vi "Write YSI Data X.vi"(0 "Output File":path=path "c:/junk.dat", 5 "Absolute Depth In":sgl format="%.2f", 7 "Zeroed Pressure":dbl format="%.2f", 9 "YSI Array":dbl[](array[numeric]) format="%.2f", 11 "Update Pressure = False\nUpdate YSI = True":bool) -> ()   [LabVIEW 2016]
uses:
  <vilib>/Utility/file.llb/Read From Spreadsheet File (DBL).vi
  <vilib>/Utility/file.llb/Write To Spreadsheet File (DBL).vi
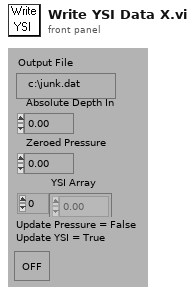
[diagram p1: front panel]
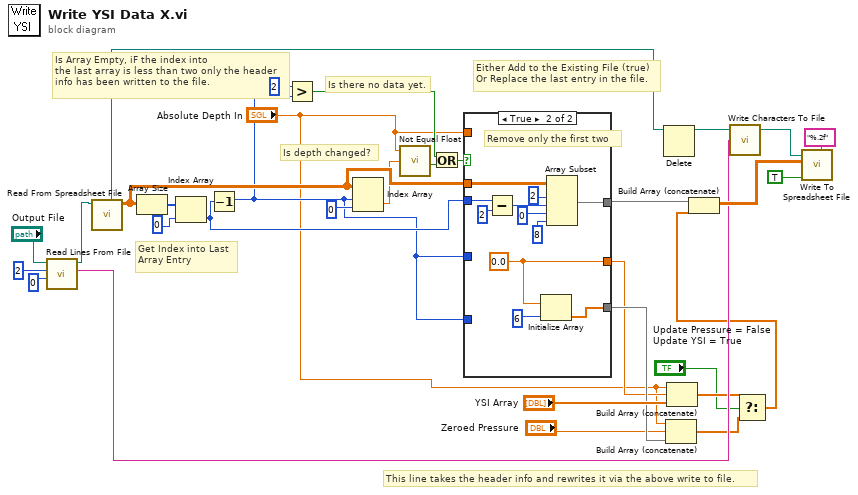
[diagram p0: block diagram]
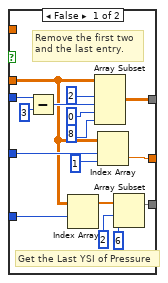
[diagram p2: hidden frame]
diagram:
  # "Is there no data yet."
  # "This line takes the header info and rewrites it via the above write to file."
  # "Either Add to the Existing File (true)\nOr Replace the last entry in the file."
  # "Get Index into Last \nArray Entry"
  # "Is depth changed?"
  # "Is Array Empty, iF the index into\nthe last array is less than two only the header\ninfo has been written to the file."
  n1 = call <vilib>:"Read Lines From File.vi"("file path (dialog if empty)"="Output File", "number of lines (all:-1)"=2, "start of read offset (chars.:0)"=0) -> ("new file path (Not A Path if cancelled)"=w14:path, "line string"=w16:string)  [unwired: 3 in, 2 out]
  n2 = call-poly <vilib>:"Read From Spreadsheet File.vi"("file path (dialog if empty)"=w14) -> ("all rows"=w23:dbl[][], "new file path (Not A Path if cancelled)"=w13:path)  [unwired: 6 in, 3 out]
  n3 = Array Size(array=w23) -> (size(s)=w32:i32[])
  n4 = Index Array(array=w32, index=0) -> (element=w12:i32)
  n5 = Decrement(x=w12) -> (x-1=w11:i32)
  n6 = Greater?(x=2, y=w11) -> (0:w25:bool)
  n7 = Index Array(array=w23, index (row)=w11, index (col)=0) -> (element=w1:dbl)
  n8 = call "Not Equal Float.vi"("Input 2"=w1, "Input 1"="Absolute Depth In") -> ("Not Equal"=w27:bool)  [unwired: 1 in]
  n9 = Or(x=w25, y=w27) -> (x .or. y?=w26:bool)
  n10 = case shown="True" w26 {
    tunnel: w23 -> [w38 w59]
    tunnel: w11 -> [w40 _]
    tunnel: "Absolute Depth In" -> [_ _]
    tunnel: [w48 w58] -> w22
    tunnel: [w44 w51] -> w8
    tunnel: w12 -> [w39 w52]
    tunnel: [w36 w49] -> w9
    tunnel: w11 -> [w37 _]
    frame False {
      # "Get the Last YSI of Pressure"
      # "Remove the first two\nand the last entry."
      n11 = Subtract(x=w39, y=3) -> (x-y=w41:i32)
      n12 = Index Array(array=w38, index (row)=w37) -> (element=w35:dbl[])  [unwired: 1 in]
      n13 = Array Subset(array=w38, index (row)=2, length (row)=w41, index (col)=0, length (col)=8) -> (w48:dbl[][])
      n14 = Index Array(array=w38, index (row)=w40, index (col)=1) -> (element=w44:dbl)
      n15 = Array Subset(array=w35, index=2, length=6) -> (w36:dbl[])
    }
    frame True {
      w51 = 0.0
      # "Remove only the first two"
      n16 = Subtract(x=w52, y=2) -> (x-y=w56:i32)
      n17 = Initialize Array(w51, 6) -> (w49:dbl[])
      n18 = Array Subset(array=w59, index (row)=2, length (row)=w56, index (col)=0, length (col)=8) -> (w58:dbl[][])
    }
  }
  n19 = Delete(path (use dialog)=w13) -> (deleted path=w17:path)  [unwired: 4 in, 2 out]
  n20 = Build Array (concatenate)("Absolute Depth In", "Zeroed Pressure", w9) -> (w5:dbl[])
  n21 = Build Array (concatenate)("Absolute Depth In", w8, "YSI Array") -> (w6:dbl[])
  n22 = call <vilib>:"Write Characters To File.vi"("character string"=w16, "file path (dialog if empty)"=w17) -> ("new file path (Not A Path if cancelled)"=w18:path)  [unwired: 3 in]
  n23 = Select(t=w6, s="Update Pressure = False\nUpdate YSI = True", f=w5) -> (s? t:f=w4:dbl[])
  n24 = Build Array (concatenate)(w22, w4) -> (w24:dbl[][])
  n25 = call-poly <vilib>:"Write To Spreadsheet File.vi"("format (%.3f)"="%.2f", "append to file? (new file:F)"=TRUE, "2D data"=w24, "file path (dialog if empty)"=w18) -> ()  [unwired: 4 in, 1 out]
